vi "Destroy Message Transport.vi"(8 "error in":errorcluster, 11 "IMessageTransport in":refnum<class "IMessageTransport.lvclass">) -> (0 "error out":errorcluster, 3 "IMessageTransport out":refnum<class "IMessageTransport.lvclass">)   [LabVIEW 2016, in "IMessageTransport.lvclass"]
uses:
  IMessageTransport.lvclass
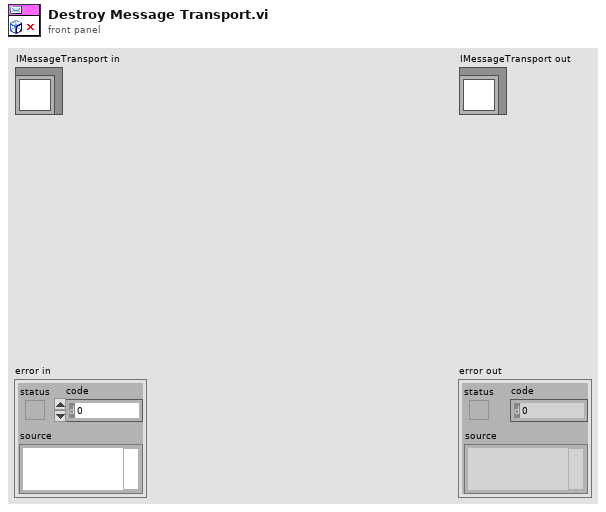
[diagram p1: front panel]
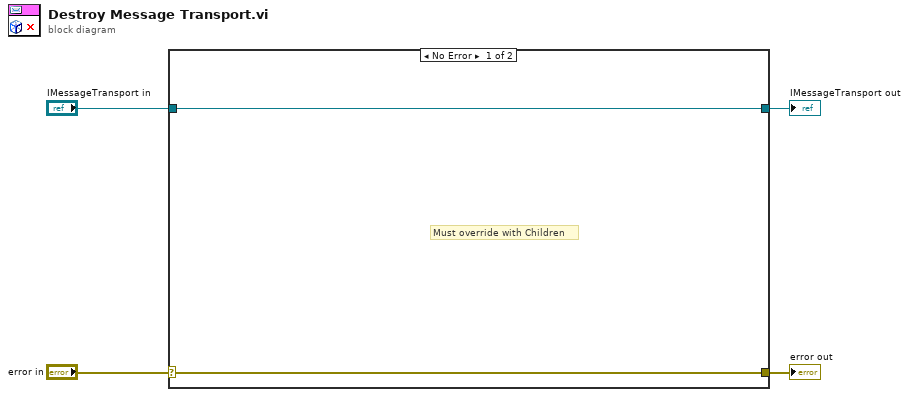
[diagram p0: block diagram]
diagram:
  n1 = case shown="No Error" "error in" {
    selector: "error in" -> [w5 w8]
    tunnel: [w5 w8] -> w3
    tunnel: [w6 w7] -> w1
    tunnel: "IMessageTransport in" -> [w6 w7]
    frame No Error {
      # "Must override with Children"
    }
    frame Error {
    }
  }
  "error out" <- w3
  "IMessageTransport out" <- w1
